vi "third.vi"() -> ()   [LabVIEW 2019]
panel:
  out "x+y":dbl
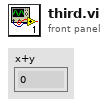
[diagram p1: front panel]
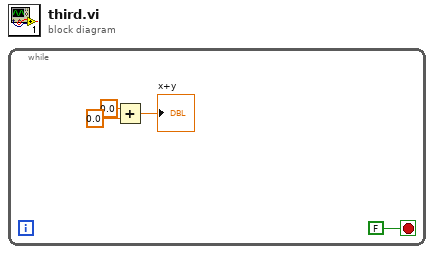
[diagram p0: block diagram]
diagram:
  n1 = while {
    stop <- FALSE stop-if-true
    n2 = Add(x=0.0, y=0.0) -> (x+y=→"x+y":dbl)
  }
